vi "read_testr.vi"() -> ()   [LabVIEW 2018]
uses:
  type.ctl
  MatFileLib.lvlib
panel:
  out "content's names":string[](array[string])
  out "number of content":i32
  out "data 3":dbl
  out "data 2":i16[][](array[numeric])
  out "data":dbl[][](array[numeric])
  out "data type":T1[](array[typedef])
  out "Contents":variant[](array[variant])
  in  "file_name":string="test1"
  in  "file path (use dialog)":path
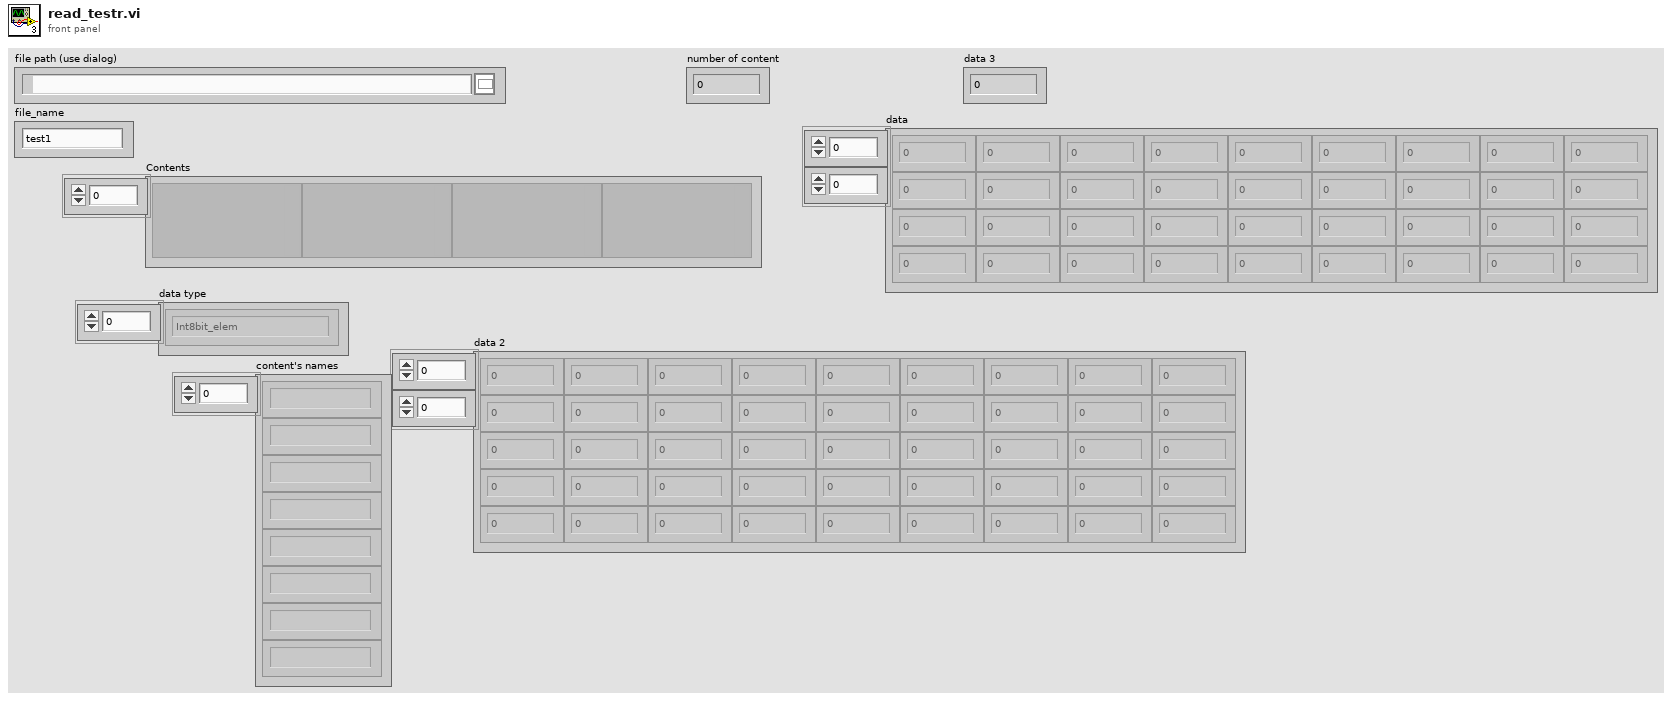
[diagram p1: front panel]
types:
  T1 = typedef "MatFileLib.lvlib/type.ctl" = enum16{"Int8bit_elem", "Int8bit", "Int64bit_elem", "Int64bit", "Int16bit_elem", "Double64bit_elem", "Int16bit", "Double64bit"}
  T2 = enum16{"open", "replace", "create", "open or create", "replace or create", "replace or create with confirmation"}
  T3 = typedef "MatFileLib.lvlib/matFile_info.ctl" = cluster{"file path (use dialog)":path, "refnum file":refnum<file>, "intermediate array":cluster{"intermediate":refnum<file>, "array name dim":i32, "row":i32, "col":i32, "Content":string, "Enum":T1}[]}
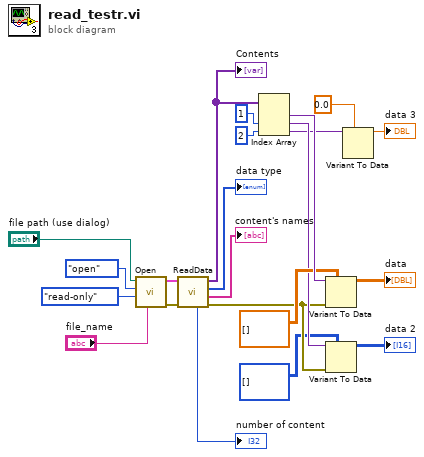
[diagram p0: block diagram]
diagram:
  n1 = call "Open.vi"("file_name"="file_name", "access (0:read/write)"=enum16{"read/write", "read-only", "write-only"}."read-only", "operation (0:open)"=T2."open", "file path (use dialog)"="file path (use dialog)") -> ("error out"=w19:errorcluster, "matFile_info"=w18:T3)  [unwired: 5 in]
  n2 = call "ReadData.vi"("error in"=w19, "matFile_info"=w18) -> ("error out"=w9:errorcluster, "content's names"=→"content's names":string[], "data type"=→"data type":T1[], "contents"=w15:variant[], "number of content"=→"number of content":i32)  [unwired: 5 in]
  "Contents" <- w15
  n3 = Index Array(array=w15, index #2=1 ("index"), index #3=2 ("index")) -> (element #1=w14:variant, element #2=w10:variant, element #3=w5:variant)  [unwired: 1 in]
  n4 = Variant To Data(error in=w9, type=dbl[][] [], Variant=w14) -> (data=→"data":dbl[][])  [unwired: 1 out]
  n5 = Variant To Data(error in=w9, type=i16[][] [], Variant=w10) -> (data=→"data 2":i16[][])  [unwired: 1 out]
  n6 = Variant To Data(type=0.0, Variant=w5) -> (data=→"data 3":dbl)  [unwired: 1 in, 1 out]
